vi "Menuactions.vi"(8 "Name":string, 10 "ItemTag":string, 11 "Default in":T1) -> (0 "Close?":bool, 2 "Name out":string, 3 "Default out":T1)   [LabVIEW 2016]
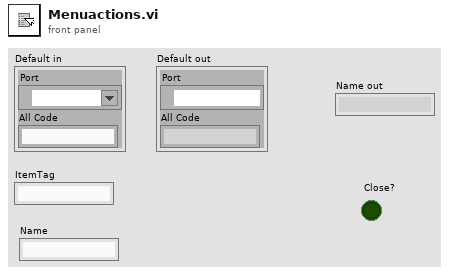
[diagram p1: front panel]
types:
  T1 = cluster{"Port":refnum<visa-resource-name>, "All Code":string}
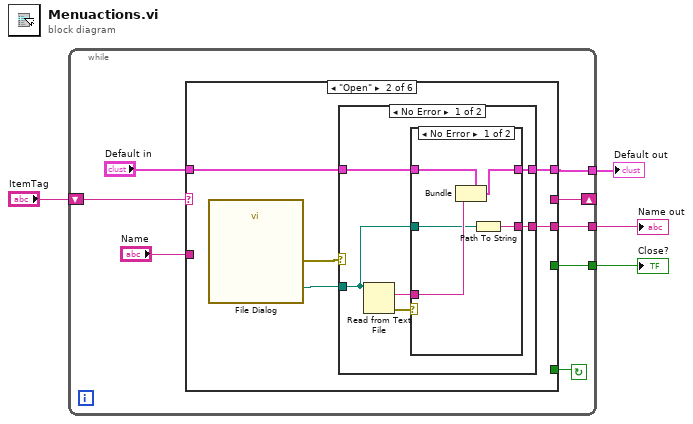
[diagram p0: block diagram]
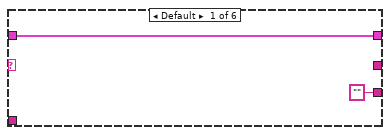
[diagram p2: hidden frame]
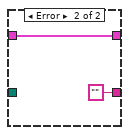
[diagram p3: hidden frame]
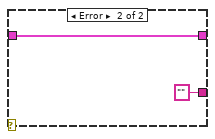
[diagram p4: hidden frame]
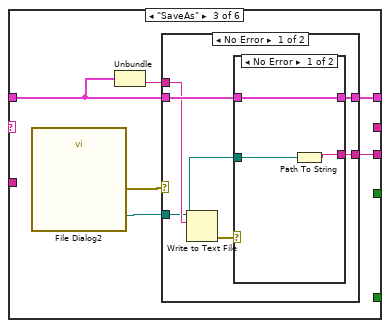
[diagram p5: hidden frame]
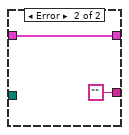
[diagram p6: hidden frame]
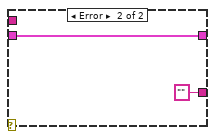
[diagram p7: hidden frame]
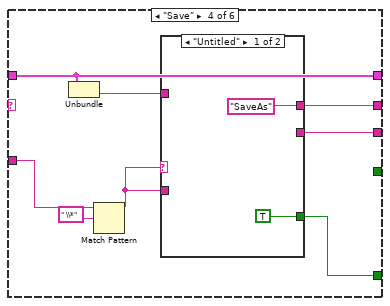
[diagram p8: hidden frame]
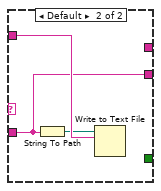
[diagram p9: hidden frame]
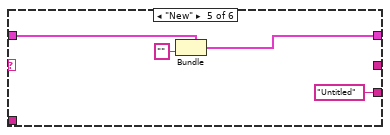
[diagram p10: hidden frame]
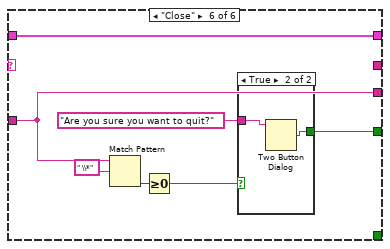
[diagram p11: hidden frame]
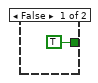
[diagram p12: hidden frame]
diagram:
  n1 = while {
    tunnel: [w12] -> w4
    shift-right: [w6] -> _
    shift-left: "ItemTag" -> [w10]
    tunnel: [w7] -> w2
    tunnel: [w5] -> w1
    stop <- w8 continue-if-true
    n2 = case shown="\"Open\"" w10 {
      tunnel: "Default in" -> [w14 w17 w37 w61 w70 w77]
      tunnel: [w14 w16 w38 w61 w68 w77] -> w12
      tunnel: "Name" -> [_ _ _ w55 _ w71]
      tunnel: [_ _ _ w58 _ _] -> w8
      tunnel: [_ _ _ _ _ w75] -> w7
      tunnel: [_ _ _ w59 _ _] -> w6
      tunnel: ["" ("Name") w15 w35 w57 "Untitled" ("Name") w71] -> w5
      frame Default {
      }
      frame "Open" {
        n3 = call "File Dialog"() -> ("selected path"=w19:path, "error out"=w18:errorcluster)  [unwired: 12 in, 2 out]
        n4 = case shown="No Error" w18 {
          tunnel: w19 -> [w21 _]
          tunnel: w17 -> [w24 w34]
          tunnel: [w22 w34] -> w16
          tunnel: [w20 ""] -> w15
          frame No Error {
            n5 = Read from Text File(file (use dialog)=w21) -> (text=w23:string, error out=w25:errorcluster)  [unwired: 3 in, 2 out]
            n6 = case shown="No Error" w25 {
              tunnel: w24 -> [w30 w32]
              tunnel: w23 -> [w29 _]
              tunnel: [w28 w32] -> w22
              tunnel: w21 -> [w27 _]
              tunnel: [w26 ""] -> w20
              frame No Error {
                n7 = Bundle(cluster=w30, "All Code"=w29) -> (w28:T1)  [unwired: 1 in]
                n8 = Path To String(path=w27) -> (string=w26:string)
              }
              frame Error {
              }
            }
          }
          frame Error {
          }
        }
      }
      frame "SaveAs" {
        n9 = call "File Dialog2"() -> ("selected path"=w40:path, "error out"=w39:errorcluster)  [unwired: 12 in, 2 out]
        n10 = Unbundle(w37) -> ("All Code"=w36:string)  [unwired: 1 out]
        n11 = case shown="No Error" w39 {
          tunnel: w40 -> [w42 _]
          tunnel: w37 -> [w45 w53]
          tunnel: [w44 w53] -> w38
          tunnel: w36 -> [w43 _]
          tunnel: [w41 ""] -> w35
          frame No Error {
            n12 = Write to Text File(file (use dialog)=w42, text=w43) -> (error out=w46:errorcluster)  [unwired: 2 in, 2 out]
            n13 = case shown="No Error" w46 {
              tunnel: w45 -> [w49 w51]
              tunnel: [w49 w51] -> w44
              tunnel: w42 -> [w48 _]
              tunnel: [w47 ""] -> w41
              frame No Error {
                n14 = Path To String(path=w48) -> (string=w47:string)
              }
              frame Error {
              }
            }
          }
          frame Error {
          }
        }
      }
      frame "Save" {
        n15 = Unbundle(w61) -> ("All Code"=w60:string)  [unwired: 1 out]
        n16 = Match Pattern(string=w55, regular expression=" \\*" ("string")) -> (before substring=w54:string)  [unwired: 1 in, 3 out]
        n17 = case shown="\"Untitled\"" w54 {
          tunnel: w54 -> [_ w64]
          tunnel: w60 -> [_ w66]
          tunnel: ["SaveAs" _] -> w59
          tunnel: [TRUE _] -> w58
          tunnel: [_ w64] -> w57
          frame "Untitled" {
          }
          frame Default {
            n18 = String To Path(string=w64) -> (path=w65:path)
            n19 = Write to Text File(file (use dialog)=w65, text=w66) -> ()  [unwired: 2 in, 3 out]
          }
        }
      }
      frame "New" {
        n20 = Bundle(cluster=w70, "All Code"="") -> (w68:T1)  [unwired: 1 in]
      }
      frame "Close" {
        n21 = Match Pattern(string=w71, regular expression=" \\*" ("string")) -> (offset past match=w74:i32)  [unwired: 1 in, 3 out]
        n22 = Greater Or Equal To 0?(x=w74) -> (x >= 0?=w72:bool)
        n23 = case shown="True" w72 {
          tunnel: "Are you sure you want to quit?" ("message") -> [_ w80]
          tunnel: [TRUE ("T button?") w79] -> w75
          frame False {
          }
          frame True {
            n24 = Two Button Dialog(message=w80) -> (T button?=w79:bool)  [unwired: 2 in]
          }
        }
      }
    }
  }
  "Default out" <- w4
  "Close?" <- w2
  "Name out" <- w1
